vi "Read Suggestion IO.vi"(8 "error in (no error)":errorcluster, 11 "IntelliSenseStringControl in":refnum<class "IntelliSenseStringControl.lvclass">) -> (0 "error out":errorcluster, 2 "Suggestion IO":refnum<class "SuggestionIObase.lvclass">, 3 "IntelliSenseStringControl out":refnum<class "IntelliSenseStringControl.lvclass">)   [LabVIEW 2016, in "StringIntelliSense.lvlib" / "IntelliSenseStringControl.lvclass"]
uses:
  IntelliSenseStringControl.lvclass
  Suggestions IO/base/SuggestionIObase.lvclass
  IntelliSenseStringControl.lvclass/IntelliSenseStringControl.ctl
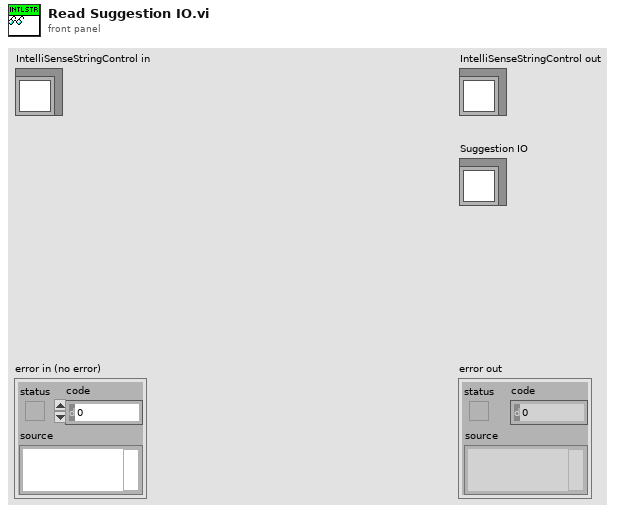
[diagram p1: front panel]
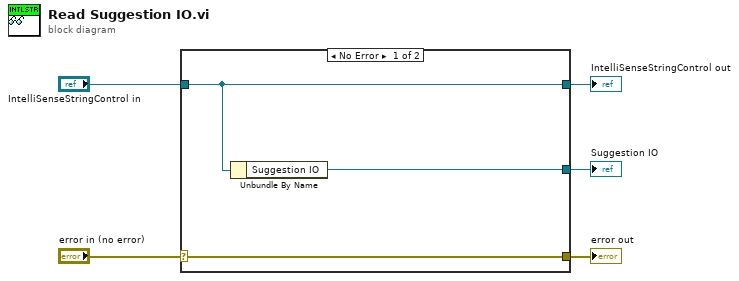
[diagram p0: block diagram]
diagram:
  n1 = case shown="No Error" "error in (no error)" {
    selector: "error in (no error)" -> [w8 w9]
    tunnel: [w8 w9] -> w4
    tunnel: [w7 w10] -> w2
    tunnel: "IntelliSenseStringControl in" -> [w7 w10]
    tunnel: [w6 _] -> w1
    frame No Error {
      n2 = Unbundle By Name(w7) -> ("Suggestion IO"=w6:refnum<class "SuggestionIObase.lvclass">)
    }
    frame Error {
    }
  }
  "error out" <- w4
  "IntelliSenseStringControl out" <- w2
  "Suggestion IO" <- w1
